vi "9000 Not implemented--error.vi"(8 "error in":errorcluster) -> (0 "error out":errorcluster)   [LabVIEW 2020, in "SDO Manager.lvlib" / "SDO Manager.lvclass"]
uses:
  SDO Manager.lvclass
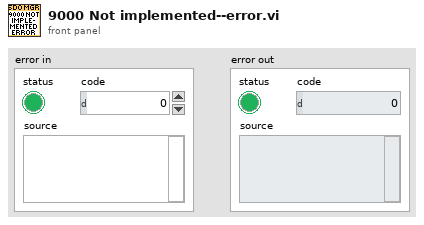
[diagram p1: front panel]
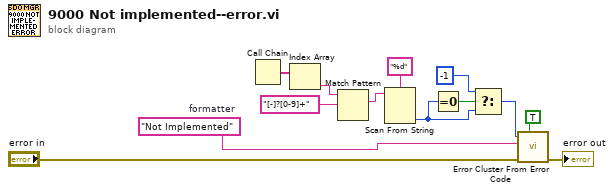
[diagram p0: block diagram]
diagram:
  w1 = "Not Implemented"  # formatter
  n1 = Call Chain() -> (call chain=w4:string[])
  n2 = Index Array(array=w4) -> (element=w9:string)  [unwired: 1 in]
  n3 = Match Pattern(string=w9, regular expression="[-]?[0-9]+") -> (match substring=w10:string)  [unwired: 1 in, 3 out]
  n4 = Scan From String(format string="%d", input string=w10) -> (output 1=w6:i32)  [unwired: 3 in, 3 out]
  n5 = Equal To 0?(x=w6) -> (x = 0?=w7:bool)
  n6 = Select(t=-1, s=w7, f=w6) -> (s? t:f=w3:i32)
  n7 = call <vilib>:"Error Cluster From Error Code.vi"("show call chain? (False)"=TRUE, "error in (no error)"="error in", "error message (\"\")"=w1, "error code (0)"=w3) -> ("error out"=→"error out":errorcluster)  [unwired: 5 in]
